vi "Log Path.vi"() -> (2 "Log File Reference":refnum<file>)   [LabVIEW 2015]
uses:
  <vilib>/Utility/sysdir.llb/System Directory Type.ctl
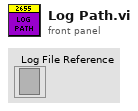
[diagram p1: front panel]
types:
  T1 = enum16{"open", "replace", "create", "open or create", "replace or create", "replace or create with confirmation"}
  T2 = typedef "System Directory Type.ctl" = i32
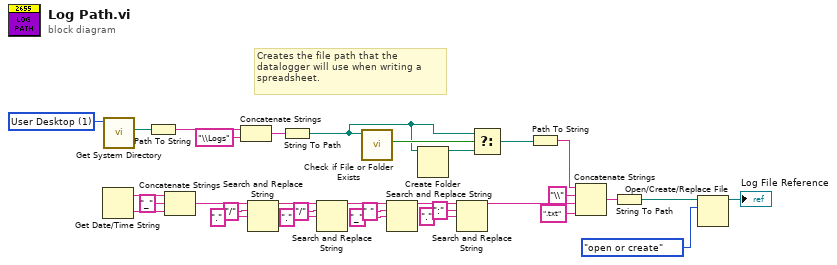
[diagram p0: block diagram]
diagram:
  w14 = T2 1 items=["User Home"=0, "User Desktop"=1, "User Documents"=2, "User Application Data"=3, "User Preferences"=4, "User Temporary"=5, "Public Documents"=6, "Public Application Data"=7, "Public Preferences"=8, "Public Cache"=13, "System Core Libraries"=9, "System Installed Libraries"=10, "Application Files"=11, "Boot Volume Root"=12] ("system directory type")
  # "Creates the file path that the datalogger will use when writing a spreadsheet."
  n1 = Get Date/Time String() -> (date string=w32:string, time string=w31:string)  [unwired: 3 in]
  n2 = call <vilib>:"Get System Directory.vi"("system directory type"=w14) -> ("system directory"=w13:path)  [unwired: 10 in]
  n3 = Path To String(path=w13) -> (string=w8:string)
  n4 = Concatenate Strings(w32, "_" ("string"), w31) -> (w18:string)
  n5 = Concatenate Strings(w8, "\\Logs") -> (w6:string)
  n6 = Search and Replace String(input string=w18, search string="/", replace string="." ("replace string (\"\")")) -> (result string=w27:string)  [unwired: 5 in, 3 out]
  n7 = String To Path(string=w6) -> (path=w1:path)
  n8 = Search and Replace String(input string=w27, search string="/", replace string="." ("replace string (\"\")")) -> (result string=w24:string)  [unwired: 5 in, 3 out]
  n9 = call <vilib>:"Check if File or Folder Exists.vi"("path"=w1) -> ("file or folder exists?"=w3:bool)  [unwired: 8 in, 2 out]
  n10 = Search and Replace String(input string=w24, search string=" ", replace string="_" ("replace string (\"\")")) -> (result string=w21:string)  [unwired: 5 in, 3 out]
  n11 = Create Folder(path (use dialog)=w1) -> (created path=w2:path)  [unwired: 2 in, 2 out]
  n12 = Search and Replace String(input string=w21, search string=":", replace string="." ("replace string (\"\")")) -> (result string=w12:string)  [unwired: 5 in, 3 out]
  n13 = Select(t=w1, s=w3, f=w2) -> (s? t:f=w4:path)
  n14 = Path To String(path=w4) -> (string=w5:string)
  n15 = Concatenate Strings(w5, "\\" ("string"), w12, ".txt" ("string")) -> (w17:string)
  n16 = String To Path(string=w17) -> (path=w10:path)
  n17 = Open/Create/Replace File(file path (use dialog)=w10, operation (0:open)=T1."open or create") -> (refnum out=→"Log File Reference":refnum<file>)  [unwired: 4 in, 2 out]
